vi "Sender Actor.vi"(9 "Self Attributes":T1, 10 "Relation":T3=enum."Creator", 11 "Msg in":refnum<class "Msg.lvclass">) -> (3 "Msg out":refnum<class "Msg.lvclass">)   [LabVIEW 2021, in "jettl.lvlib" / "Msg.lvclass"]
uses:
  Msg.lvclass
  Sender/Relation.ctl
  Actor/Attributes.ctl
  Actor/Implemented Msgs.ctl
  Sender/Sender/Sender.lvclass
  Sender/Sender.lvlib
  Actor/Actor.lvlib
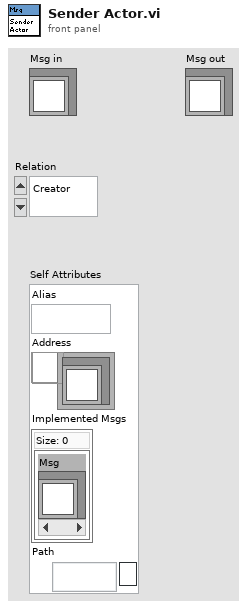
[diagram p1: front panel]
types:
  T1 = typedef "jettl.lvlib/Actor.lvlib/Attributes.ctl" = cluster{"Alias":string, "Address":refnum<user-event>, "Implemented Msgs":T2, "Path":path}
  T2 = typedef "jettl.lvlib/Actor.lvlib/Implemented Msgs.ctl" = set{refnum<class "Msg.lvclass">}
  T3 = typedef "jettl.lvlib/Sender.lvlib/Relation.ctl" = enum16{"Self", "Creator", "Created"}
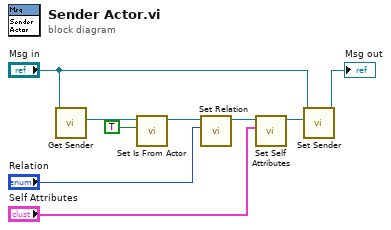
[diagram p0: block diagram]
diagram:
  n1 = call-dynamic "Get Sender.vi"("Msg in"="Msg in") -> ("Sender"=w6:refnum<class "Sender.lvclass">)  [unwired: 10 in]
  n2 = call-dynamic "Set Is From Actor.vi"("Is From Actor"=TRUE, "Sender in"=w6) -> ("Sender out"=w3:refnum<class "Sender.lvclass">)  [unwired: 9 in]
  n3 = call-dynamic "Set Relation.vi"("Relation"="Relation", "Sender in"=w3) -> ("Sender out"=w2:refnum<class "Sender.lvclass">)  [unwired: 9 in]
  n4 = call-dynamic "Set Self Attributes.vi"("Self Attributes"="Self Attributes", "Sender in"=w2) -> ("Sender out"=w4:refnum<class "Sender.lvclass">)  [unwired: 9 in]
  n5 = call-dynamic "Set Sender.vi"("Sender"=w4, "Msg in"="Msg in") -> ("Msg out"=→"Msg out":refnum<class "Msg.lvclass">)  [unwired: 9 in]
